vi "Motor Output.vi"(7 "Max Power":dbl=1.0, 9 "Backward":bool, 10 "Forward":bool, 11 "Motor refnum name":string) -> (2 "Motor Output":dbl)   [LabVIEW 2013]
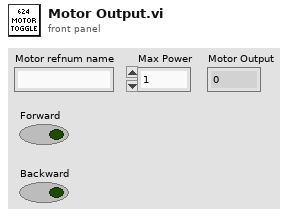
[diagram p1: front panel]
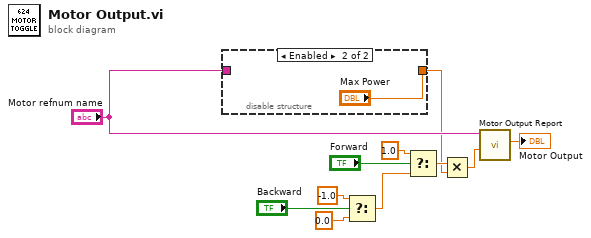
[diagram p0: block diagram]
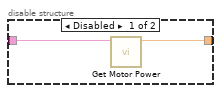
[diagram p2: hidden frame]
diagram:
  n1 = disable-structure shown="Enabled" {
    disable-tunnel: "Motor refnum name" -> [w13 _]
    disable-tunnel: [w12 "Max Power"] -> w2
    frame Disabled {
      n2 = call "Get Motor Power.vi"("Motor refnum name"=w13) -> ("Max Power"=w12:dbl)  [unwired: 10 in]
    }
    frame Enabled {
    }
  }
  n3 = Select(t=-1.0, s="Backward", f=0.0) -> (s? t:f=w9:dbl)
  n4 = Select(t=1.0, s="Forward", f=w9) -> (s? t:f=w5:dbl)
  n5 = Multiply(x=w5, y=w2) -> (x*y=w4:dbl)
  n6 = call "Motor Output Report.vi"("Motor Speed"=w4, "Motor refnum name"="Motor refnum name") -> ("Motor Output"=→"Motor Output":dbl)  [unwired: 9 in]
